vi "Write System Configuration.vi"(8 "error in":errorcluster, 10 "System Configuration":refnum<class "PL_System Configuration.lvclass">, 11 "SystemConfigRepo in":refnum<class "SystemConfigRepo.lvclass">) -> (0 "error out":errorcluster, 3 "SystemConfigRepo out":refnum<class "SystemConfigRepo.lvclass">)   [LabVIEW 2013, in "PL Framework Configuration Tool.lvlib" / "SystemConfigRepo.lvclass"]
uses:
  SystemConfigRepo.lvclass
  Framework Configuration Classes/system configuration/PL_System Configuration.lvclass
  SystemConfigRepo.lvclass/SystemConfigRepo.ctl
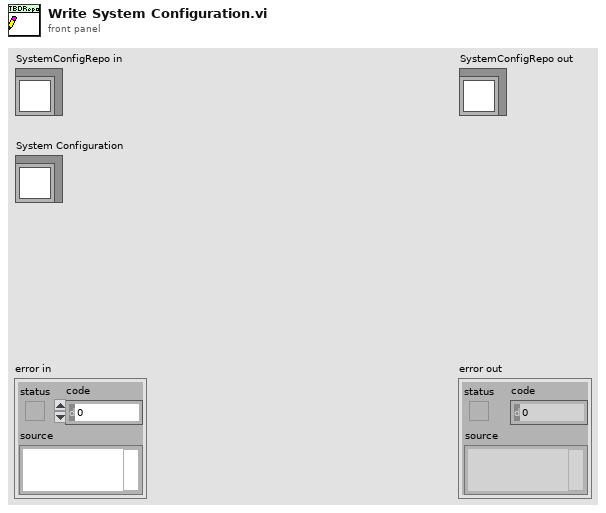
[diagram p1: front panel]
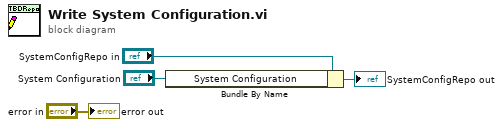
[diagram p0: block diagram]
diagram:
  n1 = Bundle By Name(cluster="SystemConfigRepo in", "System Configuration"="System Configuration") -> (→"SystemConfigRepo out":refnum<class "SystemConfigRepo.lvclass">)
  "error out" <- "error in"
